vi "SA_PREAMP.vi"(0 "VISA resource name":refnum<visa-resource-name>="TCPIP0::169.254.70.120::inst0::INSTR", 2 "IsPSA?(t)":bool, 11 "error in (no error)":errorcluster, 13 "Internal Preamp (0: Off)":i32(ring)=2 items=["Off", "Low Band", "Full Range"]) -> (4 "VISA resource name out":refnum<visa-resource-name>="TCPIP0::169.254.70.120::inst0::INSTR", 15 "error out":errorcluster)   [LabVIEW 2018]
doc: "Configures Preselector, Internal Preamp and Max Mixer Level."
uses:
  Initialize References/Station References Global.vi
  Keysight N9010A/Agilent MXA Series/Agilent MXA Series.lvlib
panel:
  out "WR(CMD)":string
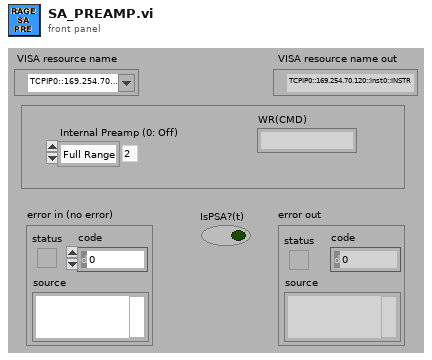
[diagram p1: front panel]
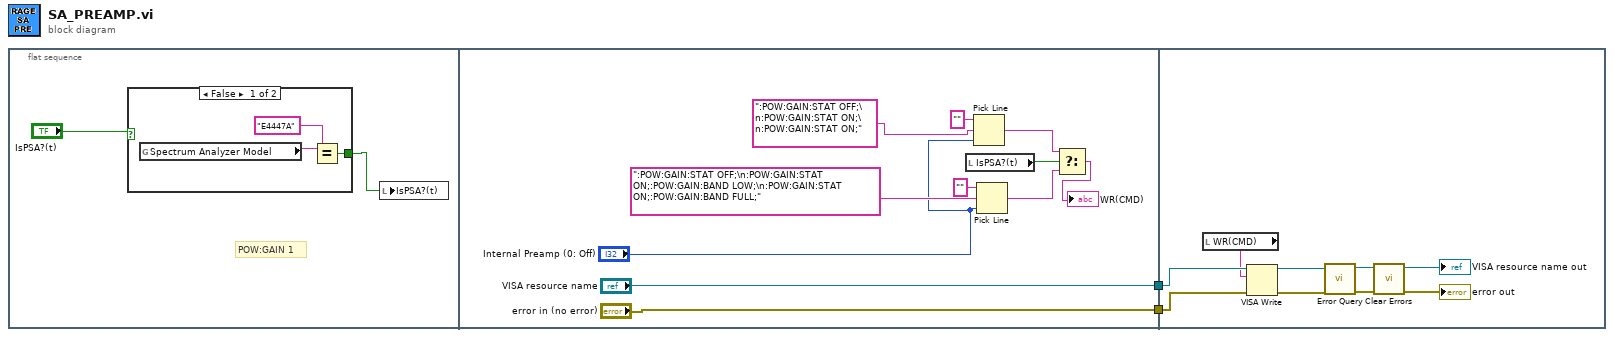
[diagram p0: block diagram]
diagram:
  n1 = flat-sequence {
    tunnel: ["VISA resource name"] -> w2
    tunnel: ["error in (no error)"] -> w1
    tunnel: w2 -> [w21]
    tunnel: w1 -> [w22]
    frame #0 {
      # "POW:GAIN 1"
      n2 = case shown="False" "IsPSA?(t)" {
        selector: "IsPSA?(t)" -> [_ w8]
        tunnel: [w5 w8] -> w4
        frame False {
          n3 = global read "Station References Global.vi" "Spectrum Analyzer Model"() -> (w7:string)
          n4 = Equal?(x=w7, y="E4447A") -> (x = y?=w5:bool)
        }
        frame True {
        }
      }
      n5 = local write "IsPSA?(t)"(w4) -> ()
    }
    frame #1 {
      n6 = local read "IsPSA?(t)"() -> (w11:bool)
      n7 = Pick Line(string ("")="", multi-line string=":POW:GAIN:STAT OFF;\n:POW:GAIN:STAT ON;\n:POW:GAIN:STAT ON;", line index="Internal Preamp (0: Off)") -> (output string=w13:string)
      n8 = Pick Line(string ("")="", multi-line string=":POW:GAIN:STAT OFF;\n:POW:GAIN:STAT ON;:POW:GAIN:BAND LOW;\n:POW:GAIN:STAT ON;:POW:GAIN:BAND FULL;", line index="Internal Preamp (0: Off)") -> (output string=w10:string)
      n9 = Select(t=w13, s=w11, f=w10) -> (s? t:f=→"WR(CMD)":string)
    }
    frame #2 {
      n10 = local read "WR(CMD)"() -> (w20:string)
      n11 = VISA Write(VISA resource name=w21, write buffer=w20, error in (no error)=w22) -> (VISA resource name out=w24:refnum<visa-resource-name>, error out=w23:errorcluster)  [unwired: 1 out]
      n12 = call "Error Query.vi"("error in (no error)"=w23, "VISA resource name"=w24) -> ("error out"=w26:errorcluster, "VISA resource name out"=→"VISA resource name out":refnum<visa-resource-name>)  [unwired: 6 in, 2 out]
      n13 = call <vilib>:"Clear Errors.vi"("error in (no error)"=w26) -> ("error out"=→"error out":errorcluster)  [unwired: 5 in, 1 out]
    }
  }
